vi "DisplayPower.vi"() -> ()   [LabVIEW 2009]
panel:
  out "Current":dbl[](graph) caption="Source Data"
  in  "Current Array":dbl[](array[numeric])
  in  "stop":bool
  out "Power":dbl[](graph) caption="Source Data"
  out "Voltage At FPGA":dbl[](graph)
  in  "Voltage Array":dbl[](array[numeric])
  in  "Power Array":dbl[](array[numeric])
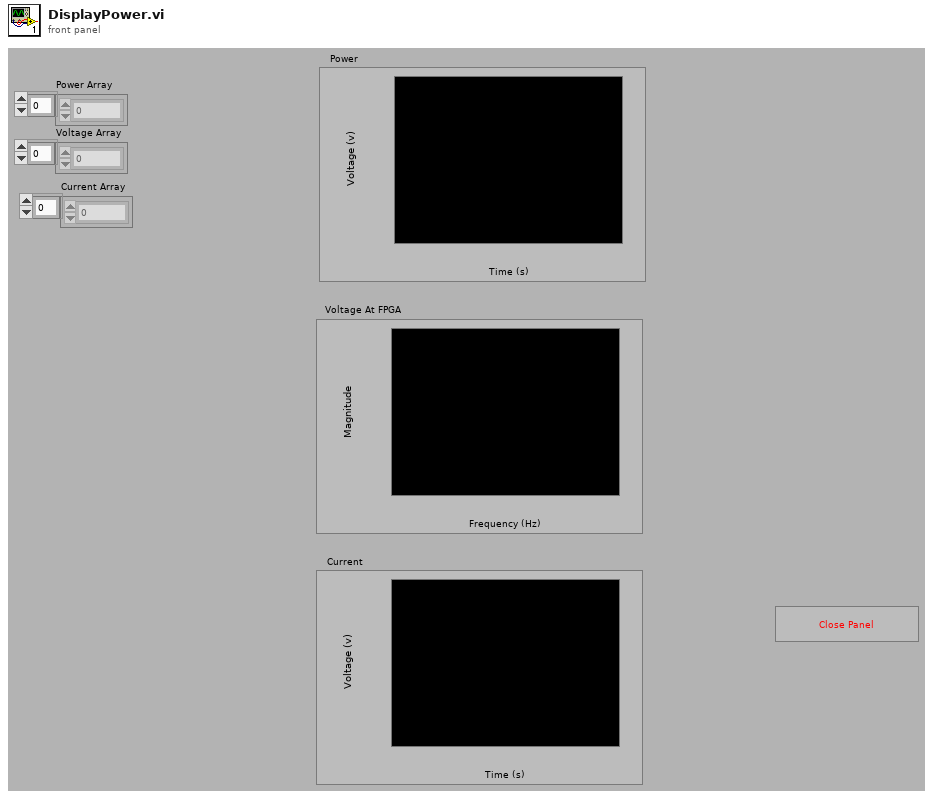
[diagram p1: front panel]
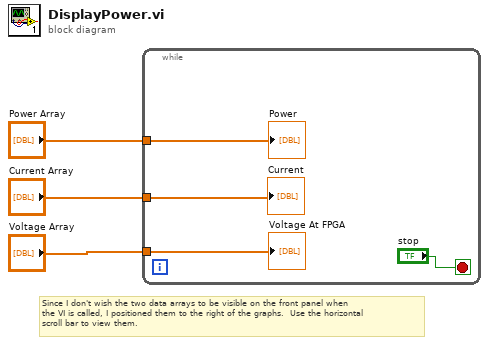
[diagram p0: block diagram]
diagram:
  # "Since I don't wish the two data arrays to be visible on the front panel when\nthe VI is called, I positioned them to the right of the graphs.  Use the horizontal\nscroll bar to view them."
  n1 = while {
    tunnel: "Current Array" -> [w7]
    tunnel: "Power Array" -> [w6]
    tunnel: "Voltage Array" -> [w5]
    stop <- "stop" stop-if-true
    "Voltage At FPGA" <- w5
    "Power" <- w6
    "Current" <- w7
  }
